vi "MFAInit.vi"() -> (0 "error out":errorcluster, 1 "Homing":bool, 2 "Timeout":bool, 3 "reference out":refnum<visa-resource-name>)   [LabVIEW 2018]
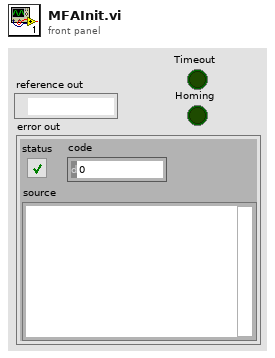
[diagram p1: front panel]
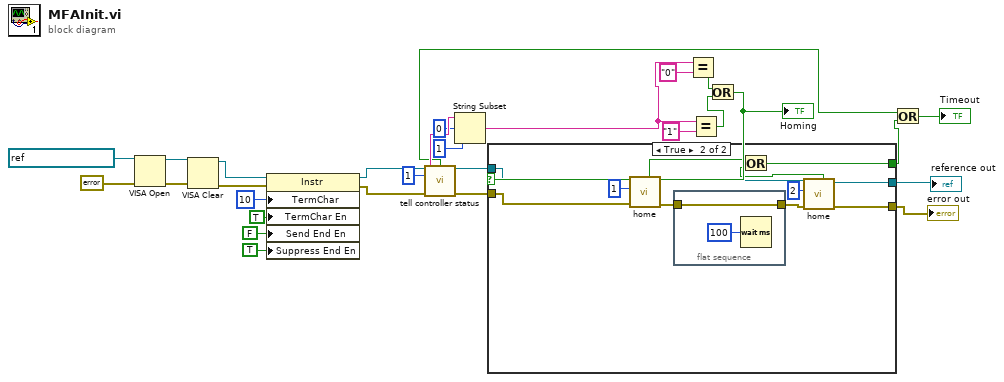
[diagram p0: block diagram]
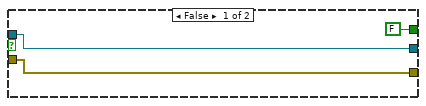
[diagram p2: hidden frame]
diagram:
  n1 = VISA Open(error in (no error)=errorcluster {"status"=FALSE, "code"=0, "source"=""}, VISA resource name=refnum<visa-resource-name> "MFAController") -> (VISA resource name=w3:refnum<visa-resource-name>, error out=w4:errorcluster)  [unwired: 3 in]
  n2 = VISA Clear(VISA resource name=w3, error in (no error)=w4) -> (VISA resource name out=w2:refnum<visa-resource-name>, error out=w1:errorcluster)
  n3 = property class="Instr"(reference=w2, error in=w1, "TermChar"=u8 10 ("Message Based Settings:Termination Character"), "TermChar En"=TRUE ("Message Based Settings:Termination Character Enable"), "Send End En"=FALSE ("Message Based Settings:Send End Enable"), "Suppress End En"=TRUE ("Message Based Settings:Suppress End Enable")) -> (reference out=w22:refnum<visa-resource-name>, error out=w23:errorcluster)
  n4 = call "tell controller status.vi"("VISA Handle in"=w22, "Axis in"=1, "error in"=w23) -> ("TimeoutFlag"=w7:bool, "VISA Handle out"=w11:refnum<visa-resource-name>, "Controller's state"=w20:string, "error out"=w10:errorcluster)  [unwired: 7 in, 2 out]
  n5 = String Subset(string=w20, offset (0)=0, length (rest)=1 ("length (rest)")) -> (substring=w15:string)
  n6 = Equal?(x=w15, y="0") -> (x = y?=w13:bool)
  n7 = Equal?(x=w15, y="1") -> (x = y?=w14:bool)
  n8 = Or(x=w13, y=w14) -> (x .or. y?=w12:bool)
  "Homing" <- w12
  n9 = case shown="True" w12 {
    tunnel: w11 -> [w32 w38]
    tunnel: w10 -> [w31 w39]
    tunnel: [w31 w37] -> w9
    tunnel: [w32 w36] -> w8
    tunnel: [FALSE w33] -> w6
    frame False {
    }
    frame True {
      n10 = call "home.vi"("error in"=w39, "Axis in"=1, "VISA Handle in"=w38) -> ("error out"=w44:errorcluster, "VISA Handle out"=w42:refnum<visa-resource-name>, "TimeoutFlag"=w35:bool)  [unwired: 3 in, 1 out]
      n11 = flat-sequence {
        tunnel: w44 -> [w46]
        tunnel: [w46] -> w41
        frame #0 {
          n12 = Wait (ms)(milliseconds to wait=u32 100) -> ()  [unwired: 1 out]
        }
      }
      n13 = call "home.vi"("error in"=w41, "Axis in"=2, "VISA Handle in"=w42) -> ("error out"=w37:errorcluster, "VISA Handle out"=w36:refnum<visa-resource-name>, "TimeoutFlag"=w34:bool)  [unwired: 3 in, 1 out]
      n14 = Or(x=w35, y=w34) -> (x .or. y?=w33:bool)
    }
  }
  "reference out" <- w8
  "error out" <- w9
  n15 = Or(x=w7, y=w6) -> (x .or. y?=→"Timeout":bool)
